vi "CAN Talon Speed Control Encoder.vi"() -> ()   [LabVIEW 2015]
doc: "This example shows how to control motor speed using CAN Jaguar and a quadrature encoder. For details setting up and understanding CAN Jaguar, see the Can Jaguar Fundamentals tutorial accessable from the LabVIEW Getting Started Window.\n\nTo control the motor speed, a PID control loop runs on the Jaguar. Notice that the encoder is wired directly to the Jaguar. One advantage of this is that the PID control does not use resources on the roboRIO. One disadvantage is that the PID code cannot be viewed or changed. However, the control can be tuned by changing the PID Parameters.\n\nOn the diagram, notice that the PID tuning parameters are only applied once before the motor is enabled. To learn about changing PID parameters while the program is running, see the CAN Position Control Encoder example. Since the control loop runs on the Jaguar, the LabVIEW loop delay is set to a slow 100ms. In fact the only reason this loop needs to run is to send a new set speed and read the actual speed.\n\nCorrect tuning parameters for a PID controller are dependent on the complete system of the motor and the load. It will be difficult to tune this system if there is no load attached to the motor. While this example is not a PID tutorial, the following information may help in understanding how to tune your PID control system.\n\nP (proportional) depends on the present error, I (integral) on the accumulation of past errors, and D (derivative) is a prediction of future errors, based on the current rate of change. The proportional parameter (P) will reduce the rise time and will reduce, but never eliminate, the steady-state error. The integral parameter (I) will eliminate the steady-state error, but may make the transient response worse. The derivative parameter (D) will increase the stability of the system, reducing the overshoot, and improving the transient response. The effects of each parameter are summarized in a table on the front panel.\n\nThis example expects a USB cable connected from your development PC to the Type B USB Jack (next to the power input) on the roboRIO.\n\nThis example requires the Driver Station to be running with Teleoperated Enabled."
uses:
  <vilib>/Rock Robotics/WPI/CAN/TalonSRX/WPI_CANTalonSRX_APIControlMode.ctl
  <vilib>/Rock Robotics/WPI/CAN/TalonSRX/WPI_CANTalonSRX_APIFeedbackSelect.ctl
  <vilib>/Rock Robotics/WPI/MotorControl/WPI_MotorControlOpenCANTalonSRX.vi
panel:
  in  "Reverse Feedback Sensor":bool
  out "Feedback Chart":cluster{dbl, dbl}(graph)
  in  "I":dbl
  in  "Encoder Codes Per Rev":u16=360
  in  "F":dbl=0.01
  in  "D":dbl
  in  "P":dbl=1.0
  in  "Set Speed (RPM)":dbl(slide) scale=-2500.0..2500.0
  out "Actual Speed (RPM)":dbl(knob) scale=-2500.0..2500.0 scale format="%4d"
  in  "Master Device Number":u8
  in  "stop":bool
  # "Set these inputs before running."
  # "roboRIO Wiring Diagram"
  # "Tuning parameters"
  # "Slave Talon SRX"
  # "Master Talon SRX"
  # "Feed-Forward"
  # "Gnd"
  # "A"
  # "B"
  # "+5V"
  # "US Digital E4P Encoder"
  # "This can be set while running."
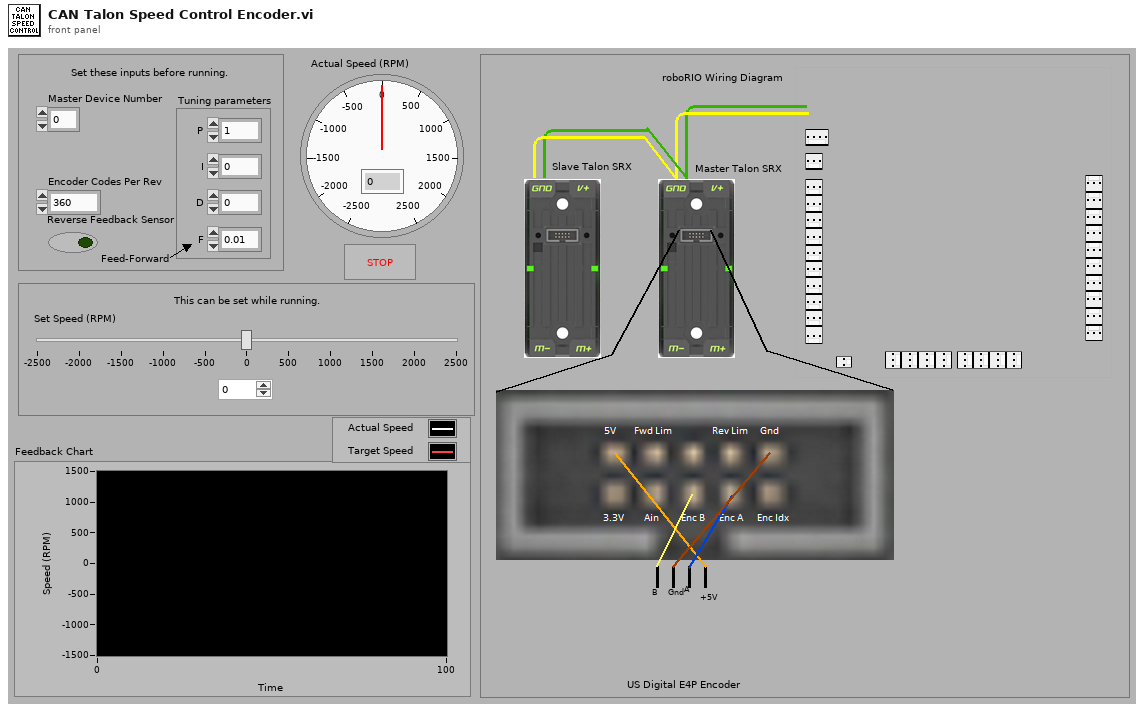
[diagram p1: front panel]
types:
  T1 = typedef "WPI_CANTalonSRX_APIFeedbackSelect.ctl" = enum16{"Digital Quadrature Encoder", "Analog Potentiometer", "Analog Encoder", "Count on Quad-A (Rising-Edge)", "Count on Quad-A (Falling-Edge)", "CTR Magnetic Enc (Absolute)", "CTR Magnetic Enc (Relative)", "Pulse Width"}
  T2 = typedef "WPI_CANTalonSRX_APIControlMode.ctl" = enum8{"Percent VBus", "Speed", "Position", "Slave", "Unchanged / Invalid", "Voltage Compensation", "Current", "Motion Profile"}
  T3 = typedef "WPI_MotorControlDeviceRef.ctl" = cluster{"DeviceStatus":errorcluster, "Type":T4, "PWM":cluster{"PWM Channel":T5, "DeadBand":T6}, "CAN":cluster{"Device Number":u8, "Control Mode":T7, "Semaphore":T8, "Max Vout":dbl, "TalonSRX Control Mode":T2}, "Invert":bool}
  T4 = typedef "WPI_MotorControlType.ctl" = enum16{"PWM", "CAN", "CANTalonSRX"}
  T5 = typedef "FPGA_DIOPWMChannel.ctl" = enum8{"PWM 0", "PWM 1", "PWM 2", "PWM 3", "PWM 4", "PWM 5", "PWM 6", "PWM 7", "PWM 8", "PWM 9", "PWM MXP 0", "PWM MXP 1", "PWM MXP 2", "PWM MXP 3", "PWM MXP 4", "PWM MXP 5", "PWM MXP 6", "PWM MXP 7", "PWM MXP 8", "PWM MXP 9", "Invalid"}
  T6 = typedef "WPI_PWMDeadband.ctl" = cluster{"Name":string, "maxPositivePwm":i32, "minPositivePwm":i32, "centerPwm":i32, "maxNegativePwm":i32, "minNegativePwm":i32, "angularRange":u16}
  T7 = typedef "WPI_CANJaguar_ControlMode.ctl" = enum8{"Percent VBus", "Current", "Speed", "Position", "Voltage"}
  T8 = typedef "Semaphore RefNum" = refnum<k1>
  T9 = typedef "WPI_CANTalonSRX_GlobalStatus.ctl" = cluster{"Applied Throttle":dbl, "Module Enabled":bool, "CAN Error":errorcluster, "Closed Loop Error":dbl, "Forward Limit Switch Closed":bool, "Reverse Limit Switch Closed":bool, "Sensor Position":dbl, "Sensor Velocity":dbl, "Current":dbl, "Sticky Fault - Over Temp":bool, "Sticky Fault - Under Voltage":bool, "Sticky Fault - Forward Limit":bool, "Sticky Fault - Reverse Limit":bool, "Sticky Fault - Forward Soft Limit":bool, "Sticky Fault - Reverse Soft Limit":bool, "Brake is Enabled":bool, "Encoder Position":dbl, "Encoder Velocity":dbl, "Encoder Index Count":dbl, "Encoder A Pin State":bool, "Encoder B Pin State":bool, "Encoder Index Pin State":bool, "Analog In":dbl, "Analog In Velocity":dbl, "Temperature (C)":dbl, "Battery Voltage":dbl, "Control 5 Is Supported":bool, "Current Profile Slot Select":dbl, "Pos Div 8":bool, "Vel Div 4":bool, "Pulse Width Position":i32, "Pulse Width Velocity":i32, "Pulse Width Rise To Rise (us)":i32, "Pulse Width Rise To Fall (us)":i32, "Mot Prof Active Is Under Run":bool, "Mot Prof Active Has Under Run":bool, "Mot Prof Active Is Last":bool, "Mot Prof Active Velocity Only":bool, "Mot Prof Active Is Valid":bool, "Mot Prof Buffer Is Full":bool, "Mot Prof Active Profile Slot Select":i32, "Mot Prof NextID":i32, "Mot Prof Count":i32, "Mot Prof Active Velocity":dbl, "Mot Prof Active Position":dbl, "Mot Prof Output Enable":i32}
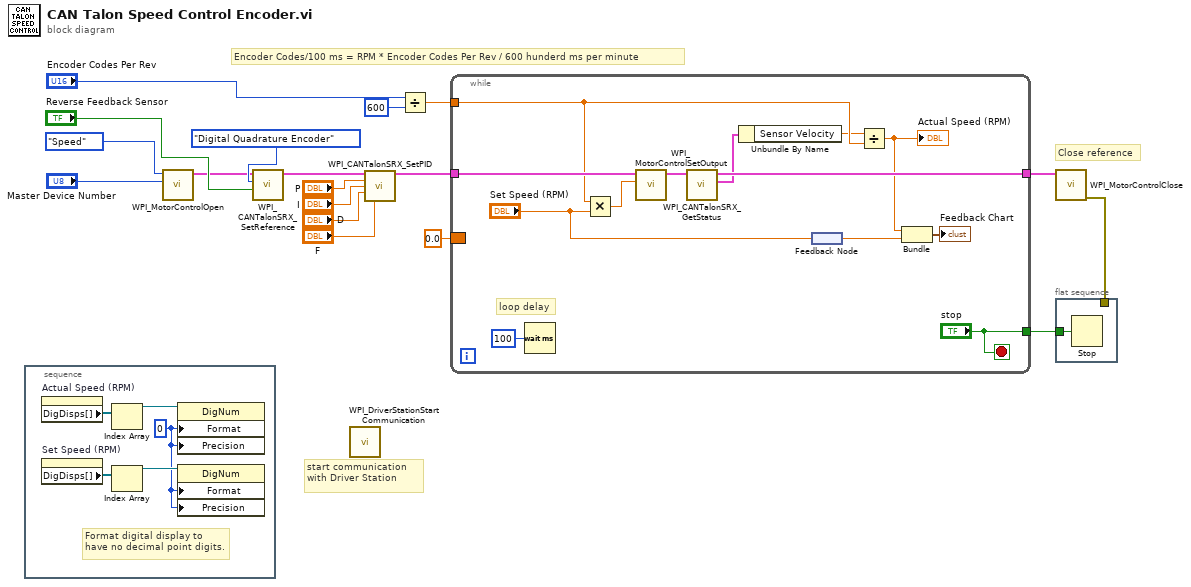
[diagram p0: block diagram]
diagram:
  # "Encoder Codes/100 ms = RPM * Encoder Codes Per Rev / 600 hunderd ms per minute"
  # "start communication with Driver Station"
  # "Close reference"
  n1 = stacked-sequence {
    frame #0 {
      w19 = u8 0 ("Display Format:Format")
      # "Format digital display to have no decimal point digits."
      n2 = property on="Actual Speed (RPM)" class="Knob (strict)"() -> ("DigDisps[]"=w23:refnum<vi>[])  [unwired: 2 in, 2 out]
      n3 = property on="Set Speed (RPM)" class="Slide (strict)"() -> ("DigDisps[]"=w20:refnum<vi>[])  [unwired: 2 in, 2 out]
      n4 = Index Array(array=w23) -> (element=w22:refnum<vi>)  [unwired: 1 in]
      n5 = Index Array(array=w20) -> (element=w21:refnum<vi>)  [unwired: 1 in]
      n6 = property class="DigNum"(reference=w22, "Format"=w19, "Precision"=w19) -> ()  [unwired: 1 in, 2 out]
      n7 = property class="DigNum"(reference=w21, "Format"=w19, "Precision"=w19) -> ()  [unwired: 1 in, 2 out]
    }
  }
  n8 = call-poly <vilib>:"WPI_MotorControlOpen.vi"("Device Number"="Master Device Number", "Control Mode"=WPI_CANTalonSRX_APIControlMode."Speed") -> ("MotorControlDeviceRef"=w4:T3)  [unwired: 3 in, 6 out]
  n9 = call <vilib>:"WPI_CANTalonSRX_SetReference.vi"("Reverse Feedback Sensor"="Reverse Feedback Sensor", "Feedback Reference"=WPI_CANTalonSRX_APIFeedbackSelect."Digital Quadrature Encoder", "CAN Talon SRX Ref"=w4) -> ("CAN Talon SRX Ref"=w3:T3)  [unwired: 7 in, 1 out]
  n10 = call <vilib>:"WPI_DriverStationStart Communication.vi"() -> ()  [unwired: 2 in, 10 out]
  n11 = call <vilib>:"WPI_CANTalonSRX_SetPID.vi"("CAN Talon SRX Ref"=w3, "P"="P", "I"="I", "D"="D", "F"="F") -> ("CAN Talon SRX Ref"=w17:T3)  [unwired: 9 in, 1 out]
  n12 = Divide(x="Encoder Codes Per Rev", y=u16 600) -> (x/y=w11:dbl)
  n13 = while {
    tunnel: ["stop"] -> w16
    tunnel: w17 -> [w34]
    tunnel: [w33] -> w18
    tunnel: w11 -> [w32]
    border: 0.0 -> [_]
    stop <- "stop" stop-if-true
    # "loop delay"
    n14 = Wait (ms)(milliseconds to wait=u32 100) -> ()  [unwired: 1 out]
    n15 = Multiply(x=w32, y="Set Speed (RPM)") -> (x*y=w28:dbl)
    n16 = call <vilib>:"WPI_MotorControlSetOutput.vi"("Output"=w28, "MotorControlDevRef"=w34) -> ("MotorControlDevRef"=w31:T3)  [unwired: 7 in, 2 out]
    n17 = call <vilib>:"WPI_CANTalonSRX_GetStatus.vi"("CAN Talon SRX Ref"=w31) -> ("Talon SRX Status"=w30:T9, "CAN Talon SRX Ref"=w33:T3)  [unwired: 8 in, 1 out]
    n18 = Unbundle By Name(w30) -> ("Sensor Velocity"=w29:dbl)
    n19 = feedback #1() -> (w26:dbl)
    n20 = feedback-in #1("Set Speed (RPM)") -> ()
    n21 = Divide(x=w29, y=w32) -> (x/y=w27:dbl)
    "Actual Speed (RPM)" <- w27
    n22 = Bundle(w27, w26) -> (→"Feedback Chart":cluster{dbl, dbl})  [unwired: 1 in]
  }
  n23 = call <vilib>:"WPI_MotorControlClose.vi"("MotorControlDevRef"=w18) -> ("error out"=w15:errorcluster)  [unwired: 10 in]
  n24 = flat-sequence {
    tunnel: w16 -> [w37]
    tunnel: w15 -> [_]
    frame #0 {
      n25 = Stop(stop? (T)=w37) -> ()
    }
  }
